vi "Filter Wheel Validate Move Command.vi"(8 "error in (no error)":errorcluster, 10 "Filter Wheel Info":T2={"Num Wheels"=0, "Filters"=[], "Invalid Combinations"=[], "Addr"="", "Name"="", "Simulate"=FALSE, "Homing Parameters"={"Direction (F: CW)"=TRUE, "Speed"=150, "Accel"=400, "Min Distance"=2700, "Short Leg"=0, "Error Cnts"=0}, "Default Speed"=1000} {"Default Speed" min=20 max=4000 step=10}, 11 "Move":T1) -> (0 "error out":errorcluster, 2 "Valid?":bool, 3 "Move dup":T1)   [LabVIEW 2021]
uses:
  FW cmd Q Move Parameters.ctl
  Filter Wheel configuration.ctl
  Filter Wheel Object/Filter Wheel Details.ctl
  Filter Wheel Arduino Control/Filter Wheel Arduino Homing cluster.ctl
  Filter Wheel Object/Filter Wheel.lvclass
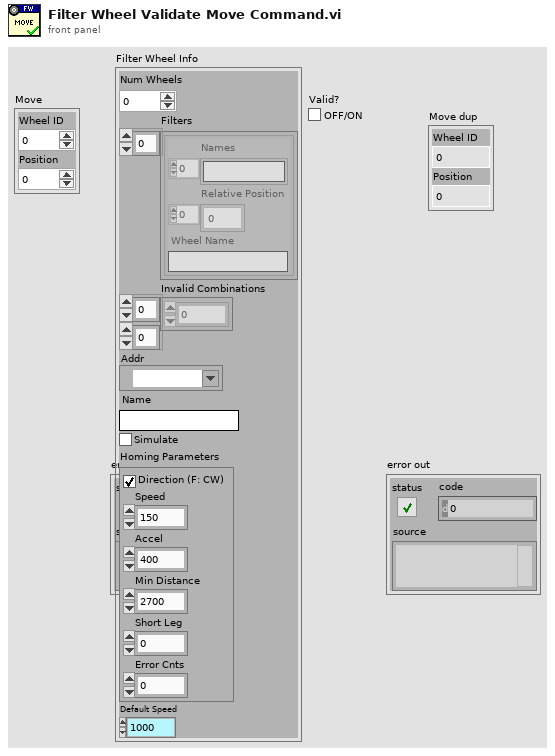
[diagram p1: front panel]
types:
  T1 = typedef "FW cmd Q Move Parameters.ctl" = cluster{"Wheel ID":i32, "Position":i32}
  T2 = typedef "Filter Wheel.lvclass/Filter Wheel configuration.ctl" = cluster{"Num Wheels":i32, "Filters":T3[], "Invalid Combinations":i32[][], "Addr":refnum<visa-resource-name>, "Name":string, "Simulate":bool, "Homing Parameters":T4, "Default Speed":u16}
  T3 = typedef "Filter Wheel.lvclass/Filter Wheel Details.ctl" = cluster{"Names":string[], "Relative Position":i32[], "Wheel Name":string}
  T4 = typedef "Filter Wheel Arduino Homing cluster.ctl" = cluster{"Direction (F: CW)":bool, "Speed":i32, "Accel":i32, "Min Distance":i32, "Short Leg":i32, "Error Cnts":i32}
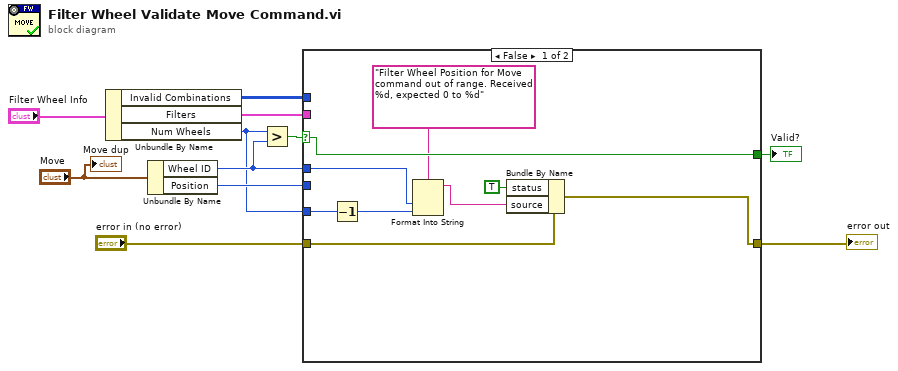
[diagram p0: block diagram]
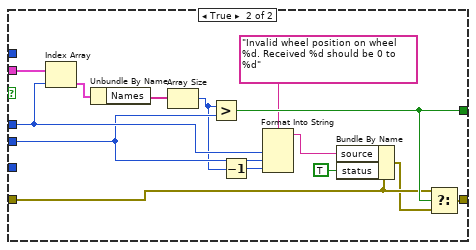
[diagram p2: hidden frame]
diagram:
  n1 = Unbundle By Name("Filter Wheel Info") -> ("Invalid Combinations"=w7:i32[][], "Filters"=w10:T3[], "Num Wheels"=w3:i32)
  n2 = Unbundle By Name("Move") -> ("Wheel ID"=w9:i32, "Position"=w6:i32)
  n3 = Greater?(x=w3, y=w9) -> (0:w8:bool)
  n4 = case shown="False" w8 {
    selector: w8 -> [w20 _]
    tunnel: w10 -> [_ w34]
    tunnel: w9 -> [w16 w25]
    tunnel: w7 -> [_ _]
    tunnel: w6 -> [_ w24]
    tunnel: [w20 w31] -> w5
    tunnel: "error in (no error)" -> [w19 w30]
    tunnel: w3 -> [w15 _]
    tunnel: [w13 w27] -> w2
    frame False {
      n5 = Decrement(x=w15) -> (x-1=w12:i32)
      n6 = Format Into String(format string="Filter Wheel Position for Move command out of range. Received %d, expected 0 to %d", w16, w12) -> (resulting string=w14:string)  [unwired: 2 in, 1 out]
      n7 = Bundle By Name(cluster=w19, "status"=TRUE, "source"=w14) -> (w13:errorcluster)
    }
    frame True {
      n8 = Index Array(array=w34, index=w25) -> (element=w33:T3)
      n9 = Unbundle By Name(w33) -> ("Names"=w32:string[])
      n10 = Array Size(array=w32) -> (size(s)=w23:i32)
      n11 = Greater?(x=w23, y=w24) -> (0:w31:bool)
      n12 = Decrement(x=w23) -> (x-1=w22:i32)
      n13 = Format Into String(format string="Invalid wheel position on wheel %d. Received %d should be 0 to %d", w25, w24, w22) -> (resulting string=w21:string)  [unwired: 2 in, 1 out]
      n14 = Bundle By Name(cluster=w30, "source"=w21, "status"=TRUE) -> (w28:errorcluster)
      n15 = Select(t=w30, s=w31, f=w28) -> (s? t:f=w27:errorcluster)
    }
  }
  "error out" <- w2
  "Valid?" <- w5
  "Move dup" <- "Move"
